vi "UpdateValueWhileTyping.vi"() -> ()   [LabVIEW 2019]
panel:
  out "StrInd":string
  in  "StrCtrl":string
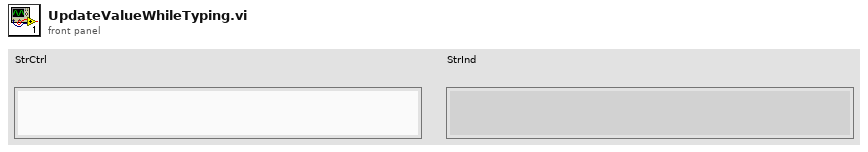
[diagram p1: front panel]
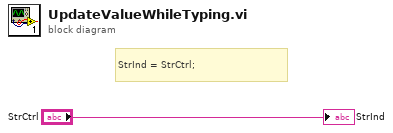
[diagram p0: block diagram]
diagram:
  # "StrInd = StrCtrl;"
  "StrInd" <- "StrCtrl"
